vi "Get Offset Tuning State.vi"(8 "error in (no error)":errorcluster, 11 "DeviceRefnum":u64) -> (0 "error out":errorcluster, 2 "Enabled?":bool, 3 "DeviceRefnum Out":u64)   [LabVIEW 2014]
doc: "Get state of the offset tuning mode"
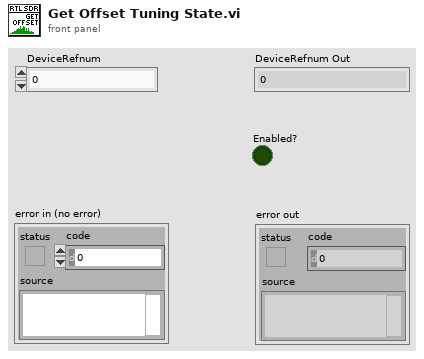
[diagram p1: front panel]
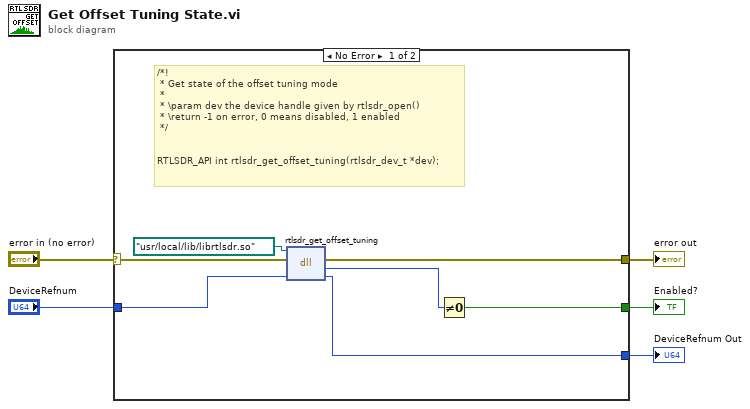
[diagram p0: block diagram]
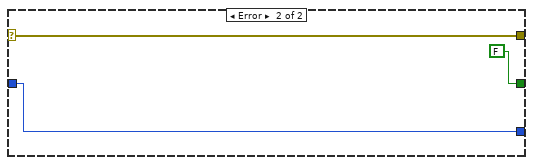
[diagram p2: hidden frame]
diagram:
  n1 = case shown="No Error" "error in (no error)" {
    selector: "error in (no error)" -> [w7 w14]
    tunnel: "DeviceRefnum" -> [w12 w15]
    tunnel: [w11 w15] -> w4
    tunnel: [w8 FALSE] -> w3
    tunnel: [w6 w14] -> w1
    frame No Error {
      # "/*!\n * Get state of the offset tuning mode\n *\n * \\param dev the device handle given by rtlsdr_open()\n * \\return -1 on error, 0 means disabled, 1 enabled\n */\n\n\nRTLSDR_API int rtlsdr_get_offset_tuning(rtlsdr_dev_t *dev);"
      n2 = dll-call lib="C:/Program Files (x86)/National Instruments/LabVIEW 2016/user.lib/rtlsdr/rtlsdr.*" fn="rtlsdr_get_offset_tuning"(path in=path "/usr/local/lib/librtlsdr.so", error in=w7, "DeviceRefnum"=w12) -> (error out=w6:errorcluster, "return type"=w9:i32, "DeviceRefnum"=w11:u64)  [unwired: 1 in, 1 out]
      n3 = Not Equal To 0?(x=w9) -> (x != 0?=w8:bool)
    }
    frame Error {
    }
  }
  "DeviceRefnum Out" <- w4
  "Enabled?" <- w3
  "error out" <- w1
